vi "sv_Compute Time to Next Optimum for Triangle Wave.vi"(7 "optimum":T1, 9 "duty cycle (50 %)":dbl, 10 "phase (0 °)":dbl, 11 "frequency (997 Hz)":dbl) -> (3 "time to optimum [s]":dbl)   [LabVIEW 2017, in "SoundVib_Generation.lvlib"]
uses:
  <vilib>/addons/_NISVFA/_Generation/SoundVib_Generation.lvlib
  <vilib>/addons/_NISVFA/_Generation/subVIs/sv_Optimum Location.ctl
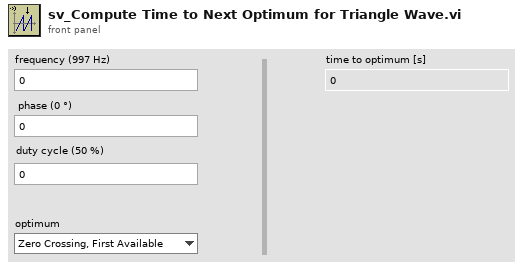
[diagram p1: front panel]
types:
  T1 = typedef "SoundVib_Generation.lvlib/sv_Optimum Location.ctl" = enum16{"Zero Crossing, First Available", "Zero Crossing, Positive Slope", "Zero Crossing, Negative Slope", "Peak or Valley", "Peak", "Valley"}
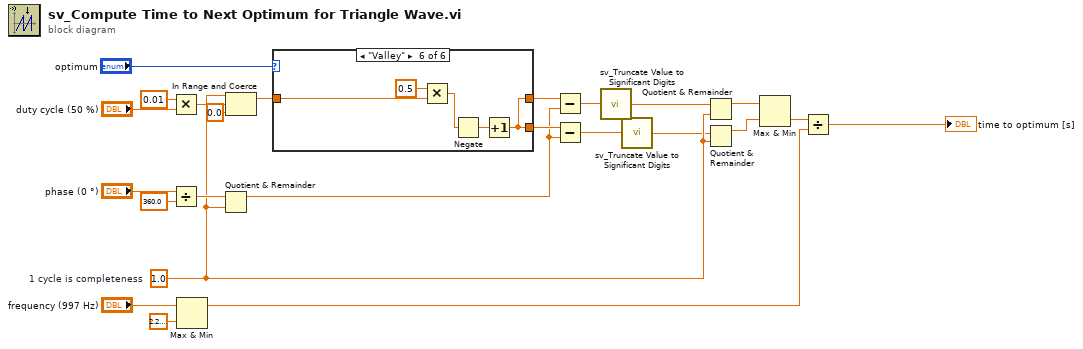
[diagram p0: block diagram]
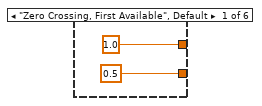
[diagram p2: hidden frame]
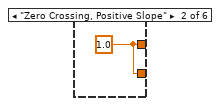
[diagram p3: hidden frame]
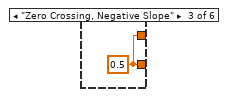
[diagram p4: hidden frame]
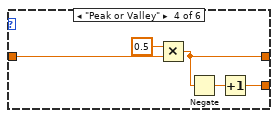
[diagram p5: hidden frame]
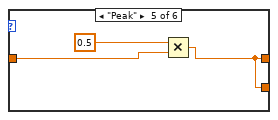
[diagram p6: hidden frame]
diagram:
  w7 = 1.0  # 1 cycle is completeness
  n1 = Multiply(x=0.01, y="duty cycle (50 %)") -> (x*y=w8:dbl)
  n2 = Divide(x="phase (0 °)", y=360.0 ("time to optimum [s]")) -> (x/y=w21:dbl)
  n3 = Max & Min(x="frequency (997 Hz)", y=2.220446049250313e-16) -> (max(x,y)=w13:dbl)  [unwired: 1 out]
  n4 = Quotient & Remainder(x=w21, y=w7) -> (x-y*floor(x/y)=w6:dbl)  [unwired: 1 out]
  n5 = In Range and Coerce(upper limit=w7, x=w8, lower limit=0.0) -> (coerced(x)=w9:dbl)  [unwired: 1 out]
  n6 = case shown="\"Valley\"" "optimum" {
    tunnel: [1.0 ("time to optimum [s]") w27 w28 w31 w34 w37] -> w12
    tunnel: [0.5 ("1 cycle is completeness") w27 w28 w30 w34 w37] -> w11
    tunnel: w9 -> [_ _ _ w33 w36 w41]
    frame "Zero Crossing, First Available", Default {
    }
    frame "Zero Crossing, Positive Slope" {
      w27 = 1.0 ("time to optimum [s]")
    }
    frame "Zero Crossing, Negative Slope" {
      w28 = 0.5 ("time to optimum [s]")
    }
    frame "Peak or Valley" {
      n7 = Multiply(x=0.5, y=w33) -> (x*y=w31:dbl)
      n8 = Negate(x=w31) -> (-x=w29:dbl)
      n9 = Increment(x=w29) -> (x+1=w30:dbl)
    }
    frame "Peak" {
      n10 = Multiply(x=0.5, y=w36) -> (x*y=w34:dbl)
    }
    frame "Valley" {
      n11 = Multiply(x=0.5, y=w41) -> (x*y=w39:dbl)
      n12 = Negate(x=w39) -> (-x=w38:dbl)
      n13 = Increment(x=w38) -> (x+1=w37:dbl)
    }
  }
  n14 = Subtract(x=w12, y=w6) -> (x-y=w4:dbl)
  n15 = Subtract(x=w11, y=w6) -> (x-y=w2:dbl)
  n16 = call <vilib>:"sv_Truncate Value to Significant Digits.vi"("value"=w4) -> ("truncated value"=w3:dbl)  [unwired: 14 in]
  n17 = call <vilib>:"sv_Truncate Value to Significant Digits.vi"("value"=w2) -> ("truncated value"=w1:dbl)  [unwired: 14 in]
  n18 = Quotient & Remainder(x=w3, y=w7) -> (x-y*floor(x/y)=w20:dbl)  [unwired: 1 out]
  n19 = Quotient & Remainder(x=w1, y=w7) -> (x-y*floor(x/y)=w19:dbl)  [unwired: 1 out]
  n20 = Max & Min(x=w20, y=w19) -> (min(x,y)=w18:dbl)  [unwired: 1 out]
  n21 = Divide(x=w18, y=w13) -> (x/y=→"time to optimum [s]":dbl)
